vi "FIB mode.vi"(5 "Close session":bool, 7 "Initialization":bool, 8 "error in":errorcluster, 9 "Iterations":u32=2, 10 "FIB mode":T1(ring)=enum."Milling", 11 "COM port in":refnum<visa-resource-name>) -> (0 "error out":errorcluster, 3 "COM port out":refnum<visa-resource-name>)   [LabVIEW 2018]
uses:
  <vilib>/Instr/_visa.llb/VISA Configure Serial Port (Instr).vi
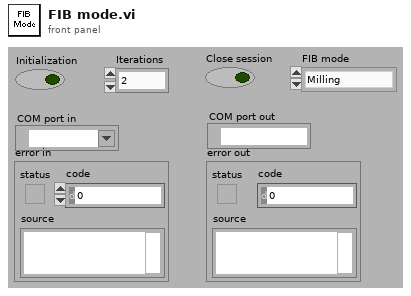
[diagram p1: front panel]
types:
  T1 = enum16{"SEM", "FIB", "Milling", "SEM + FIB", "Mill + SEM", "SEM Drift Correction", "FIB Drift Correction", "No Beam", "External", "External + SEM"}
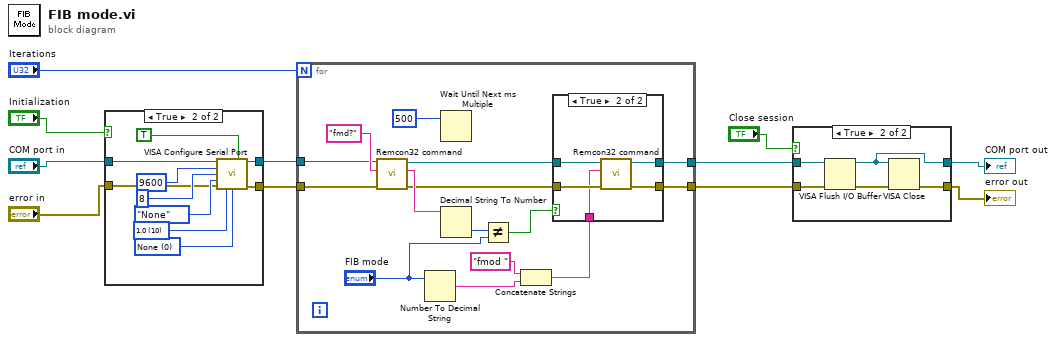
[diagram p0: block diagram]
diagram:
  n1 = case shown="True" "Initialization" {
    tunnel: [w13 w17] -> w2
    tunnel: [w12 w16] -> w1
    tunnel: "COM port in" -> [w13 w15]
    tunnel: "error in" -> [w12 w14]
    frame False {
    }
    frame True {
      w22 = u16 0 items=["None", "XON/XOFF", "RTS/CTS", "XON/XOFF & RTS/CTS", "DTR/DSR", "XON/XOFF & DTR/DSR"] ("flow control (0:none)")
      w21 = u16 10 items=["1.0"=10, "1.5"=15, "2.0"=20] ("stop bits (10: 1 bit)")
      n2 = call-poly "VISA Configure Serial Port"("VISA resource name"=w15, "Enable Termination\nChar (T)"=TRUE ("Enable Termination\nChar (T)"), "baud rate (9600)"=u32 9600, "data bits (8)"=u16 8, "parity (0:none)"=enum16{"None", "Odd", "Even", "Mark", "Space"}."None", "error in (no error)"=w14, "stop bits (10: 1 bit)"=w21, "flow control (0:none)"=w22) -> ("VISA resource name out"=w17:refnum<visa-resource-name>, "error out"=w16:errorcluster)  [unwired: 6 out]
    }
  }
  n3 = for {
    N: "Iterations" -> [_]
    tunnel: [w38] -> w9
    tunnel: [w37] -> w8
    tunnel: w2 -> [w31]
    tunnel: w1 -> [w30]
    n4 = call "Remcon32 command.vi"("error in"=w30, "SEM command"="fmd?" ("write buffer"), "COM port in"=w31) -> ("error out"=w33:errorcluster, "SEM reply"=w36:string, "COM port out"=w34:refnum<visa-resource-name>)  [unwired: 2 in, 4 out]
    n5 = Number To Decimal String(number="FIB mode") -> (decimal integer string=w25:string)  [unwired: 1 out]
    n6 = Wait Until Next ms Multiple(millisecond multiple=u32 500) -> ()  [unwired: 1 out]
    n7 = Decimal String To Number(string=w36) -> (number=w29:i32)  [unwired: 3 out]
    n8 = Not Equal?(x=w29, y="FIB mode") -> (x != y?=w28:bool)
    n9 = Concatenate Strings("fmod " ("write buffer"), w25) -> (w24:string)
    n10 = case shown="True" w28 {
      tunnel: [w40 w43] -> w38
      tunnel: [w39 w42] -> w37
      tunnel: w34 -> [w40 w45]
      tunnel: w33 -> [w39 w44]
      tunnel: w24 -> [_ w41]
      frame False {
      }
      frame True {
        n11 = call "Remcon32 command.vi"("error in"=w44, "SEM command"=w41, "COM port in"=w45) -> ("error out"=w42:errorcluster, "COM port out"=w43:refnum<visa-resource-name>)  [unwired: 2 in, 5 out]
      }
    }
  }
  n12 = case shown="True" "Close session" {
    tunnel: w9 -> [w47 w51]
    tunnel: w8 -> [w46 w49]
    tunnel: [w47 w50] -> w7
    tunnel: [w46 w52] -> w6
    frame False {
    }
    frame True {
      n13 = VISA Flush I/O Buffer(VISA resource name=w51, error in (no error)=w49) -> (VISA resource name out=w50:refnum<visa-resource-name>, error out=w48:errorcluster)  [unwired: 1 in]
      n14 = VISA Close(VISA resource name=w50, error in (no error)=w48) -> (error out=w52:errorcluster)
    }
  }
  "COM port out" <- w7
  "error out" <- w6
